vi "Numeric Indices to Excel Cell Address.vi"(10 "Row":u32, 11 "Column":u32) -> (3 "Cell Address":string)   [LabVIEW 2019, in "Open Xml.lvlib"]
uses:
  Open Xml.lvlib
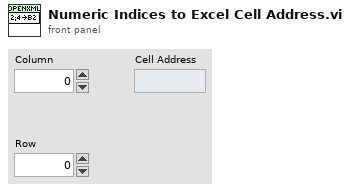
[diagram p1: front panel]
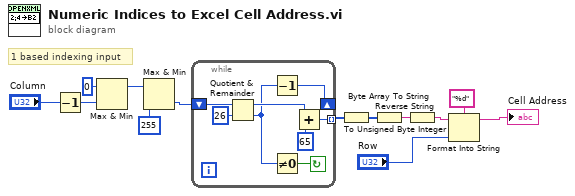
[diagram p0: block diagram]
diagram:
  # "1 based indexing input"
  n1 = Decrement(x="Column") -> (x-1=w1:u32)
  n2 = Max & Min(x=0, y=w1) -> (max(x,y)=w7:u32)  [unwired: 1 out]
  n3 = Max & Min(x=w7, y=255) -> (min(x,y)=w6:u32)  [unwired: 1 out]
  n4 = while {
    tunnel: [w18] -> w12 mode=indexing
    shift-left: w6 -> [w20]
    shift-right: [w14] -> _
    stop <- w19 continue-if-true
    n5 = Quotient & Remainder(x=w20, y=26) -> (x-y*floor(x/y)=w16:u32, floor(x/y)=w15:u32)
    n6 = Decrement(x=w15) -> (x-1=w14:u32)
    n7 = Not Equal To 0?(x=w15) -> (x != 0?=w19:bool)
    n8 = Add(x=w16, y=65) -> (x+y=w18:u32)
  }
  n9 = To Unsigned Byte Integer(number=w12) -> (unsigned 8bit integer=w11:u8[])
  n10 = Byte Array To String(unsigned byte array=w11) -> (string=w10:string)
  n11 = Reverse String(1:w10) -> (0:w9:string)
  n12 = Format Into String(format string="%d" ("Format String"), initial string=w9, "Row") -> (resulting string=→"Cell Address":string)  [unwired: 1 in, 1 out]
